vi "JYGetFW.vi"(8 "error in (no error)":errorcluster, 11 "FW RefNum In":refnum<k7>) -> (0 "error out":errorcluster, 2 "Filter Index":i32(ring)=1 items=["Filter 1"=1, "Empty"=2, "Empty"=3, "Empty"=4, "Filter 2"=5, "Filter 3"=6], 3 "FW RefNum Out":refnum<k7>)   [LabVIEW 2009]
doc: "Gets the current index position of the Filter Wheel."
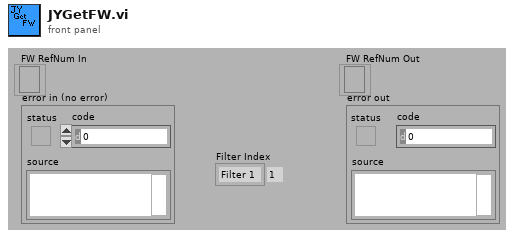
[diagram p1: front panel]
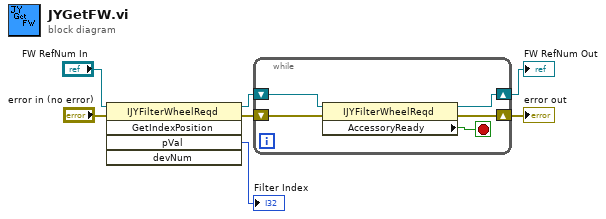
[diagram p0: block diagram]
diagram:
  n1 = invoke class="IJYFilterWheelReqd" method="GetIndexPosition"(reference="FW RefNum In", error in="error in (no error)") -> (reference out=w5:refnum<k7>, error out=w4:errorcluster, "pVal"=→"Filter Index":i32)  [unwired: 3 in, 2 out]
  n2 = while {
    shift-right: [w8] -> w2
    shift-left: w4 -> [w10]
    shift-right: [w9] -> w3
    shift-left: w5 -> [w11]
    stop <- w12 stop-if-true
    n3 = property class="IJYFilterWheelReqd"(reference=w11, error in=w10) -> (reference out=w9:refnum<k7>, error out=w8:errorcluster, "AccessoryReady"=w12:bool)
  }
  "FW RefNum Out" <- w3
  "error out" <- w2
